vi "Leds.vi"() -> ()   [LabVIEW 2022 SP3]
uses:
  <vilib>/DAQmx/write.llb/DAQmx Write (Digital 1D Bool NChan 1Samp 1Line).vi
  <vilib>/DAQmx/miscellaneous.llb/DAQmx Fill In Error Info.vi
panel:
  in  "Leds Bool":bool[](array[boolean])
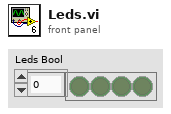
[diagram p1: front panel]
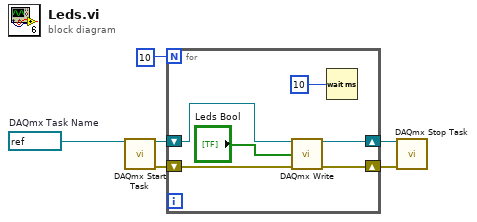
[diagram p0: block diagram]
diagram:
  w6 = refnum<k21> "LEDs"  # DAQmx Task Name
  n1 = call <vilib>:"DAQmx Start Task.vi"("task/channels in"=w6) -> ("task out"=w5:refnum<k21>, "error out"=w4:errorcluster)  [unwired: 13 in]
  n2 = for {
    N: 10 -> [_]
    shift-right: [w9] -> w3
    shift-left: w5 -> [w11]
    shift-right: [w8] -> w2
    shift-left: w4 -> [w10]
    n3 = call-poly <vilib>:"DAQmx Write.vi"("task/channels in"=w11, "data"="Leds Bool", "error in"=w10) -> ("task out"=w9:refnum<k21>, "error out"=w8:errorcluster)  [unwired: 10 in, 1 out]
    n4 = Wait (ms)(milliseconds to wait=10) -> ()  [unwired: 1 out]
  }
  n5 = call <vilib>:"DAQmx Stop Task.vi"("task/channels in"=w3, "error in"=w2) -> ()  [unwired: 12 in, 2 out]
